vi "Align Cup.vi"(2 "Top Input":dbl, 3 "Turret Angle":dbl) -> (0 "Top Output":dbl, 1 "Turret Output":dbl)   [LabVIEW 2011]
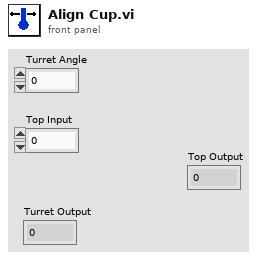
[diagram p1: front panel]
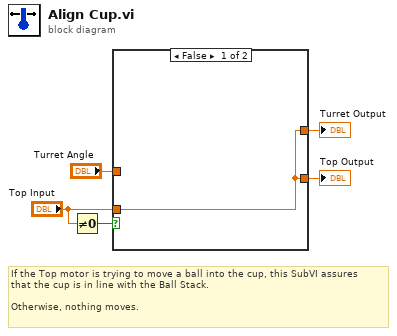
[diagram p0: block diagram]
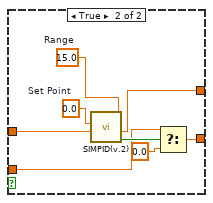
[diagram p2: hidden frame]
diagram:
  # "If the Top motor is trying to move a ball into the cup, this SubVI assures\nthat the cup is in line with the Ball Stack.\n\nOtherwise, nothing moves."
  n1 = Not Equal To 0?(x="Top Input") -> (x != 0?=w5:bool)
  n2 = case shown="False" w5 {
    tunnel: "Turret Angle" -> [_ w12]
    tunnel: [w6 w11] -> w3
    tunnel: "Top Input" -> [w6 w9]
    tunnel: [w6 w7] -> w1
    frame False {
    }
    frame True {
      w13 = 15.0  # Range
      w14 = 0.0  # Set Point
      n3 = call "SIMPID(v.2).vi"("Range"=w13, "Current Point"=w12, "Set Point"=w14) -> ("On Target"=w10:bool, "result"=w11:dbl)  [unwired: 7 in]
      n4 = Select(t=w9, s=w10, f=0.0) -> (s? t:f=w7:dbl)
    }
  }
  "Turret Output" <- w3
  "Top Output" <- w1
